vi "MES操作函数-USER.vi"(8 "error in (no error)":errorcluster caption="错误输入（无错误）", 11 "MES配置":T1={"接口地址："="http://10.9.30.175:50100/manufacturing/IntegrationServlet?InterType=XML&message=", "SITE（站点）   "="A157", "PWD（口令）"="123456", "RESOURCE（资源）"="A-6-Z-TEST", "OPERATION（工序）"="Z-TEST", "USER（用户）"="TEST", "QTY"="", "ACTIVITY"="", "NC_CODE（NG代码）"="", "启用MES"=TRUE}) -> (0 "error out":errorcluster caption="错误输出", 3 "Y":bool)   [LabVIEW 2011]
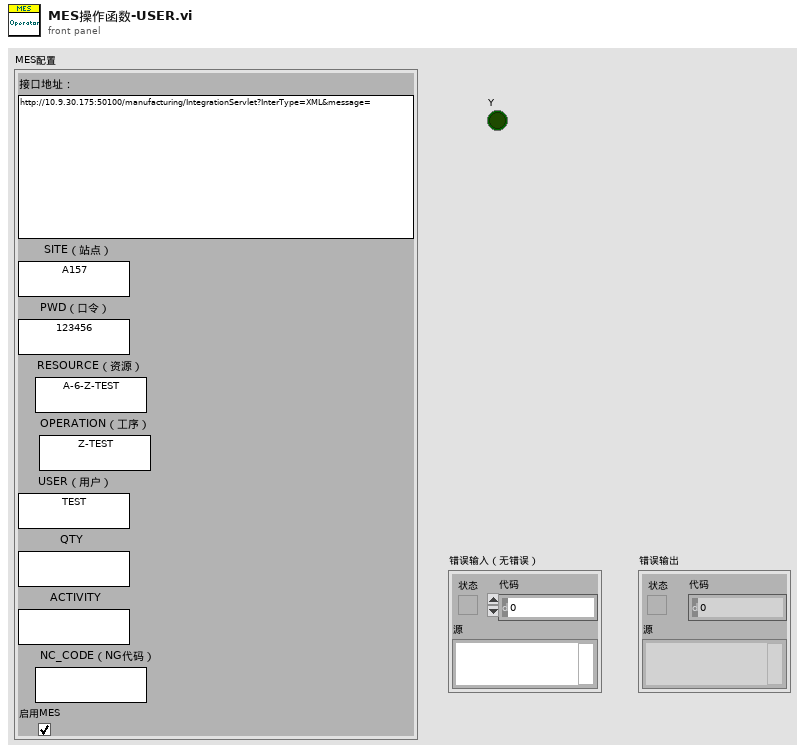
[diagram p1: front panel]
types:
  T1 = typedef "MES设置1.ctl" = cluster{"接口地址：":string, "SITE（站点）   ":string, "PWD（口令）":string, "RESOURCE（资源）":string, "OPERATION（工序）":string, "USER（用户）":string, "QTY":string, "ACTIVITY":string, "NC_CODE（NG代码）":string, "启用MES":bool}
  T2 = enum16{"USER_CHECK", "SFC_CHECK", "RLT_PASS", "RLT_ERROR", "RES_AREA"}
  T3 = cluster{"接口地址：":string, "默认值 1":i32, "接口地址：":string}
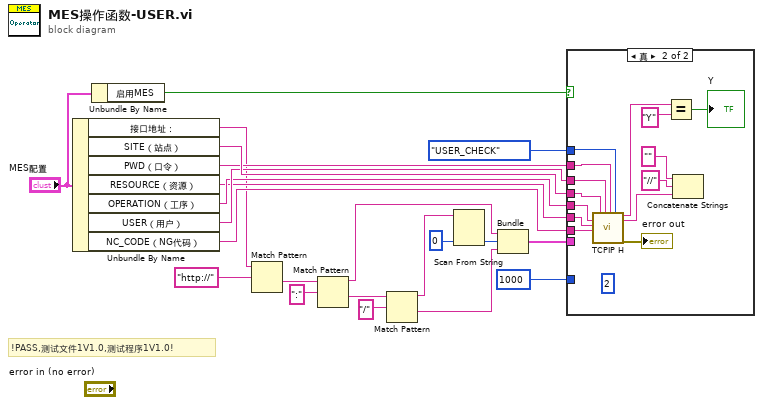
[diagram p0: block diagram]
diagram:
  # "!PASS,测试文件1V1.0,测试程序1V1.0!"
  n1 = Unbundle By Name("MES配置") -> ("接口地址："=w13:string, "SITE（站点）"=w20:string, "PWD（口令）"=w18:string, "RESOURCE（资源）"=w16:string, "OPERATION（工序）"=w17:string, "USER（用户）"=w19:string, "NC_CODE（NG代码）"=w15:string)
  n2 = Unbundle By Name("MES配置") -> ("启用MES"=w1:bool)
  n3 = Match Pattern(string=w13, regular expression="http://" ("正则表达式")) -> (after substring=w11:string)  [unwired: 1 in, 3 out]
  n4 = Match Pattern(string=w11, regular expression=":" ("正则表达式")) -> (before substring=w5:string, after substring=w9:string)  [unwired: 1 in, 2 out]
  n5 = Match Pattern(string=w9, regular expression="/" ("正则表达式")) -> (before substring=w6:string, after substring=w7:string)  [unwired: 1 in, 2 out]
  n6 = Scan From String(input string=w6, default 1=0 ("默认值 1")) -> (output 1=w3:i32)  [unwired: 3 in, 3 out]
  n7 = Bundle("接口地址："=w5, "默认值 1"=w3, "接口地址："=w7) -> (w4:T3)  [unwired: 1 in]
  n8 = case shown="真" w1 {
    tunnel: T2."USER_CHECK" ("STATE") -> [_ w36]
    tunnel: w20 -> [_ w35]
    tunnel: w19 -> [_ w34]
    tunnel: w18 -> [_ w33]
    tunnel: w17 -> [_ w32]
    tunnel: w16 -> [_ w31]
    tunnel: w15 -> [_ w30]
    tunnel: u64 1000 ("TCP超时") -> [_ _]
    tunnel: w4 -> [_ _]
    frame False {
    }
    frame True {
      (unwired) 2
      n9 = call "TCPIP H.vi"("LOT NO."=w32, "架子ID"=w31, "托盘ID+1"=w30, "作业员ID"=w35, "机器名称"=w34, "线别"=w33, "x = y?"=w36) -> ("Y&N"=w29:string, "系统消息"=w28:string, "error out"=→"error out":errorcluster)  [unwired: 8 in, 2 out]
      n10 = Equal?(x=w29, y="Y") -> (x = y?=→"Y":bool)
      n11 = Concatenate Strings("", "//" ("字符串"), w28) -> ()  [unwired: 1 out]
    }
  }
